vi "folder.vi"(7 "calling_vi":refnum<vi>, 8 "error in (no error)":errorcluster, 10 "description":string, 11 "start_path":path) -> (0 "error out":errorcluster, 3 "selected_path":path)   [LabVIEW 2015, in "lv-dialog.lvlib"]
doc: "This is identical to the file.vi using folders or the built-in file dialog, but does so for a folder using .NET. This may be more aesthetically pleasing or more obvious that you need to pick a folder and NOT a file.\n\nAlthough the input VI isn't used, it's future goal is to allow the window to be loaded on the same monitor as the VI reference wired in."
uses:
  lv-dialog.lvlib
  System.Windows.Forms
  <vilib>/Utility/error.llb/Error Cluster From Error Code.vi
  <vilib>/ErrorRing/Error Ring.xnode
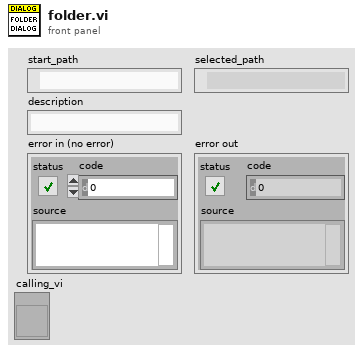
[diagram p1: front panel]
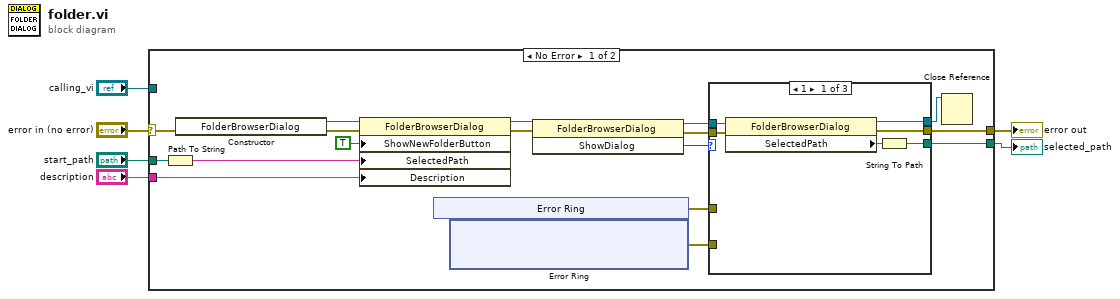
[diagram p0: block diagram]
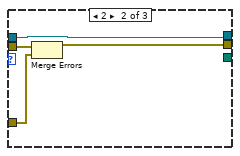
[diagram p2: hidden frame]
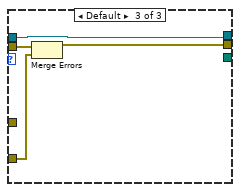
[diagram p3: hidden frame]
diagram:
  n1 = case shown="No Error" "error in (no error)" {
    selector: "error in (no error)" -> [w7 w46]
    tunnel: [w21 w46] -> w5
    tunnel: "start_path" -> [w23 _]
    tunnel: [w20 _] -> w3
    tunnel: "description" -> [w17 _]
    tunnel: "calling_vi" -> [_ _]
    frame No Error {
      n2 = Path To String(path=w23) -> (string=w22:string)
      n3 = constructor class="FolderBrowserDialog"(error in=w7) -> (reference out=w14:refnum<k24>, error out=w13:errorcluster)  [unwired: 2 in, 1 out]
      n4 = property class="FolderBrowserDialog"(reference=w14, error in=w13, "ShowNewFolderButton"=TRUE, "SelectedPath"=w22, "Description"=w17) -> (reference out=w16:refnum<k24>, error out=w15:errorcluster)
      n5 = xnode "Error Ring"() -> ("error out"=w19:errorcluster)
      n6 = xnode "Error Ring"() -> ("error out"=w18:errorcluster)
      n7 = invoke class="FolderBrowserDialog" method="ShowDialog"(reference=w16, error in=w15) -> (reference out=w10:refnum<k24>, error out=w11:errorcluster, "ShowDialog"=w9:i32)  [unwired: 1 in]
      n8 = case shown="1" w9 {
        tunnel: w10 -> [w37 w38 w42]
        tunnel: w11 -> [w36 w41 w45]
        tunnel: [w33 _ _] -> w20
        tunnel: [w35 w40 w44] -> w21
        tunnel: w19 -> [_ w39 _]
        tunnel: w18 -> [_ _ w43]
        tunnel: [w32 w38 w42] -> w8
        frame 1 {
          n9 = property class="FolderBrowserDialog"(reference=w37, error in=w36) -> (reference out=w32:refnum<k24>, error out=w35:errorcluster, "SelectedPath"=w34:string)
          n10 = String To Path(string=w34) -> (path=w33:path)
        }
        frame 2 {
          n11 = Merge Errors(w41, w39) -> (w40:errorcluster)
        }
        frame Default {
          n12 = Merge Errors(w45, w43) -> (w44:errorcluster)
        }
      }
      n13 = Close Reference(reference=w8) -> ()  [unwired: 1 in, 1 out]
    }
    frame Error {
    }
  }
  "error out" <- w5
  "selected_path" <- w3
